vi "Call Vector Field Histogram.vi"(0 "LIDAR magn. (m)":dbl[](array[numeric]), 1 "max speed":dbl=0.7, 2 "Initialize?":bool, 5 "LIDAR angle (rad)":dbl[](array[numeric]), 7 "current heading (rad)":dbl, 9 "target heading (rad)":dbl, 11 "target distance":dbl, 12 "obstacle clearance (m)":dbl, 13 "thresholds":T1) -> (4 "command vx":dbl, 6 "command vy":dbl, 8 "command heading (rad)":dbl, 10 "histogram out":dbl[](array[numeric]), 15 "mask out":bool[](array[boolean]))   [LabVIEW 2011]
uses:
  <vilib>/Analysis/coordinate.llb/Angle Rotation (scalar).vi
  <vilib>/Analysis/coordinate.llb/Wrap Angle (scalar).vi
  <vilib>/Utility/AngleManip/Degrees to Radians (Scalar DBL).vi
  <vilib>/Utility/AngleManip/Radians to Degrees (Scalar DBL).vi
  <vilib>/robotics/Obstacle Avoidance/Advanced Vector Field Histogram/NI_Robotics_Vector Field Histogram.lvlib
  <vilib>/Utility/AngleManip/NI_AngleManipulation.lvlib
  <vilib>/Analysis/NI_AAL_Angle.lvlib
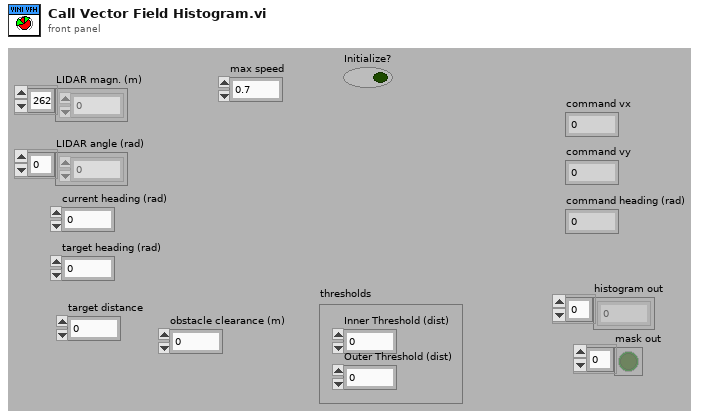
[diagram p1: front panel]
types:
  T1 = cluster{"Inner Threshold (dist)":dbl, "Outer Threshold (dist) ":dbl}
  T2 = cluster{"current heading (rad)":dbl, "target heading (rad)":dbl}
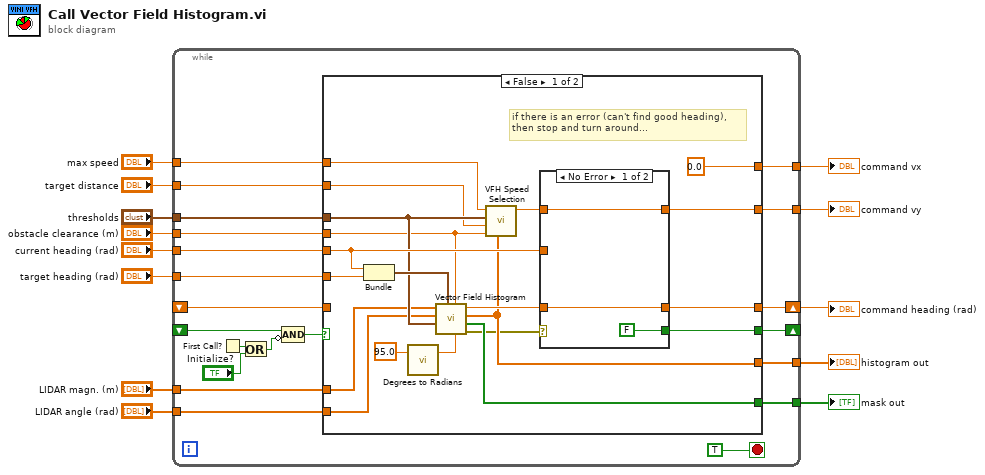
[diagram p0: block diagram]
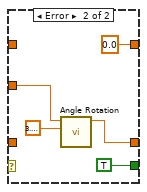
[diagram p2: hidden frame]
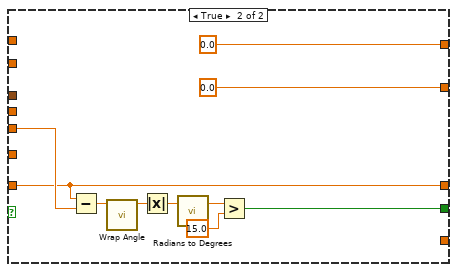
[diagram p3: hidden frame]
diagram:
  n1 = while {
    tunnel: [w33] -> w12
    tunnel: "max speed" -> [w32]
    tunnel: [w31] -> w10
    tunnel: "current heading (rad)" -> [w30]
    tunnel: [w29] -> w8
    shift-right: [w26] -> _
    shift-left: _ -> [w21]
    shift-right: [w25] -> w7
    shift-left: _ -> [w24]
    tunnel: [w34] -> w13
    tunnel: "thresholds" -> [w19]
    tunnel: "target distance" -> [w18]
    tunnel: "obstacle clearance (m)" -> [w17]
    tunnel: "target heading (rad)" -> [w16]
    tunnel: "LIDAR angle (rad)" -> [w15]
    tunnel: "LIDAR magn. (m)" -> [w14]
    stop <- TRUE stop-if-true
    n2 = First Call?() -> (First Call?: T/F=w27:bool)
    n3 = Or(x=w27, y="Initialize?") -> (x .or. y?=w22:bool)
    n4 = Compound Arithmetic op=AND(w21, invert w22) -> (w20:bool)
    n5 = case shown="False" w20 {
      tunnel: [w54 0.0 ("VX")] -> w34
      tunnel: [0.0 0.0] -> w33
      tunnel: w32 -> [w51 _]
      tunnel: [w46 _] -> w31
      tunnel: w30 -> [w47 w70]
      tunnel: [w52 _] -> w29
      tunnel: [w45 w68] -> w26
      tunnel: [w49 w67] -> w25
      tunnel: w24 -> [_ w67]
      tunnel: w19 -> [w40 _]
      tunnel: w18 -> [w39 _]
      tunnel: w17 -> [w38 _]
      tunnel: w16 -> [w37 _]
      tunnel: w15 -> [w36 _]
      tunnel: w14 -> [w35 _]
      frame False {
        # "if there is an error (can't find good heading),\nthen stop and turn around..."
        n6 = Bundle("current heading (rad)"=w47, "target heading (rad)"=w37) -> (w43:T2)  [unwired: 1 in]
        n7 = call-poly <vilib>:"Degrees to Radians.vi"("angle (deg)"=95.0) -> ("angle (rad)"=w41:dbl)  [unwired: 2 in]
        n8 = call <vilib>:"Vector Field Histogram.vi"("maximum heading change (rad)"=w41, "obstacle clearance distance"=w38, "heading"=w43, "thresholds"=w40, "direction angles (rad)"=w36, "distances"=w35) -> ("error out"=w44:errorcluster, "mask"=w52:bool[], "histogram"=w46:dbl[], "chosen heading (rad)"=w50:dbl)  [unwired: 2 in]
        n9 = call "VFH Speed Selection.vi"("Histogram"=w46, "Obstacle Clearance"=w38, "Target Distance"=w39, "Thresholds"=w40, "Max Speed"=w51) -> ("Speed"=w48:dbl)  [unwired: 6 in]
        n10 = case shown="No Error" w44 {
          tunnel: [w56 0.0 ("VX")] -> w54
          tunnel: w50 -> [w57 _]
          tunnel: [w57 w58] -> w49
          tunnel: w48 -> [w56 _]
          tunnel: w47 -> [_ w60]
          tunnel: [FALSE TRUE] -> w45
          frame No Error {
          }
          frame Error {
            n11 = call-poly <vilib>:"Angle Rotation.vi"("counterclockwise rotation"=3.141592653589793, "angle"=w60) -> ("rotated angle"=w58:dbl)  [unwired: 8 in, 1 out]
          }
        }
      }
      frame True {
        n12 = Subtract(x=w67, y=w70) -> (x-y=w64:dbl)
        n13 = call-poly <vilib>:"Wrap Angle.vi"("angle in"=w64) -> ("angle out"=w63:dbl)  [unwired: 9 in, 1 out]
        n14 = Absolute Value(x=w63) -> (abs(x)=w66:dbl)
        n15 = call-poly <vilib>:"Radians to Degrees.vi"("angle (rad)"=w66) -> ("angle (deg)"=w65:dbl)  [unwired: 2 in]
        n16 = Greater?(x=w65, y=15.0) -> (0:w68:bool)
      }
    }
  }
  "command vy" <- w13
  "command vx" <- w12
  "histogram out" <- w10
  "mask out" <- w8
  "command heading (rad)" <- w7
